vi "Get_Revision_Number.vi"() -> (0 "Revision Number":u32)   [LabVIEW 2020]
uses:
  <vilib>/Rock Robotics/Network Tables/NT Write Number.vi
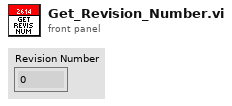
[diagram p1: front panel]
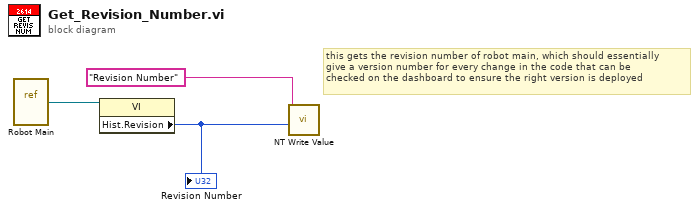
[diagram p0: block diagram]
diagram:
  # "this gets the revision number of robot main, which should essentially\ngive a version number for every change in the code that can be\nchecked on the dashboard to ensure the right version is deployed"
  n1 = vi-ref "Robot Main.vi"() -> (w1:refnum<vi>)
  n2 = property class="VI"(reference=w1) -> ("Hist.Revision"=w2:u32)  [unwired: 1 in, 2 out]
  "Revision Number" <- w2
  n3 = call-poly <vilib>:"NT Write Value.vi"("Numeric"=w2, "Name"="Revision Number") -> ()  [unwired: 9 in, 1 out]
